vi "Compare SysDef and Model Parameter File.vi"(8 "Error (in)":errorcluster, 10 "Model Parameter Filepath (.txt)":path, 11 "System Definition Filepath (.nivssdf)":path) -> (0 "Error (out)":errorcluster, 2 "Missing Parameter Lines":string[](array[string]), 3 "Missing Parameter Paths":string[](array[string]))   [LabVIEW 2016]
panel:
  out "Models":string[](array[string])
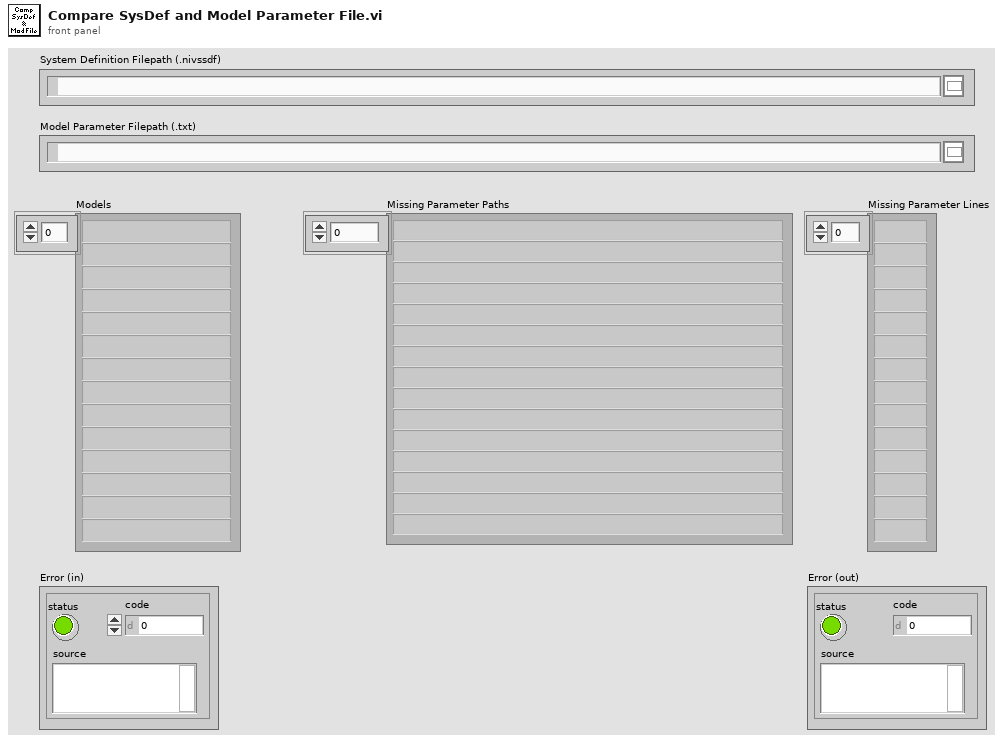
[diagram p1: front panel]
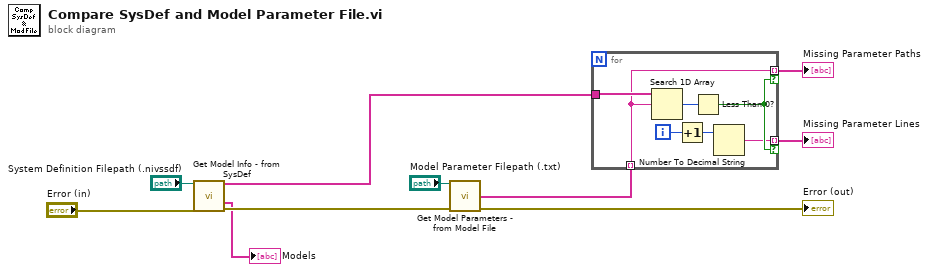
[diagram p0: block diagram]
diagram:
  n1 = call "Get Model Info - from SysDef.vi"("System Definition Filepath (.nivssdf)"="System Definition Filepath (.nivssdf)", "Error (in)"="Error (in)") -> ("Parameters"=w1:string[], "Models"=→"Models":string[], "Error (out)"=w8:errorcluster)  [unwired: 8 in, 3 out]
  n2 = call "Get Model Parameters - from Model File.vi"("Model Parameter Filepath (.txt)"="Model Parameter Filepath (.txt)", "Error (in)"=w8) -> ("Parameters"=w6:string[], "Error (out)"=→"Error (out)":errorcluster)  [unwired: 12 in]
  n3 = for {
    tunnel: w6 -> [w15] mode=indexing
    tunnel: w1 -> [w17]
    tunnel: [w15] -> w5 mode=indexing if=w14
    tunnel: [w11] -> w4 mode=indexing if=w14
    i -> [w13]
    n4 = Search 1D Array(1D array=w17, element=w15) -> (index of element=w16:i32)  [unwired: 1 in]
    n5 = Increment(x=w13) -> (x+1=w12:i32)
    n6 = Less Than 0?(x=w16) -> (x < 0?=w14:bool)
    n7 = Number To Decimal String(number=w12) -> (decimal integer string=w11:string)  [unwired: 1 in]
  }
  "Missing Parameter Paths" <- w5
  "Missing Parameter Lines" <- w4
